vi "KeithleyInit.vi"(8 "Bottom Coil (mA)":dbl, 9 "Top Coil (mA)":dbl, 11 "KeithleyVISA In":refnum<visa-resource-name>) -> (0 "error out":errorcluster, 2 "Node Out":string, 3 "KeithleyVISA Out":refnum<visa-resource-name>)   [LabVIEW 2018]
uses:
  Channel.ctl
  Keithley 2600 Series.lvlib
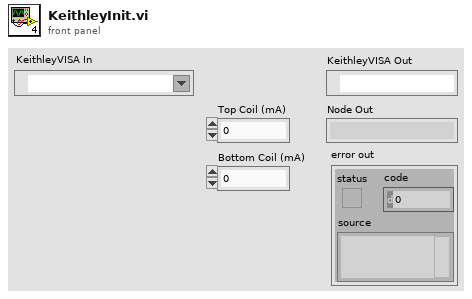
[diagram p1: front panel]
types:
  T1 = typedef "Keithley 2600 Series.lvlib/Channel.ctl" = enum32{"Channel A", "Channel B"}
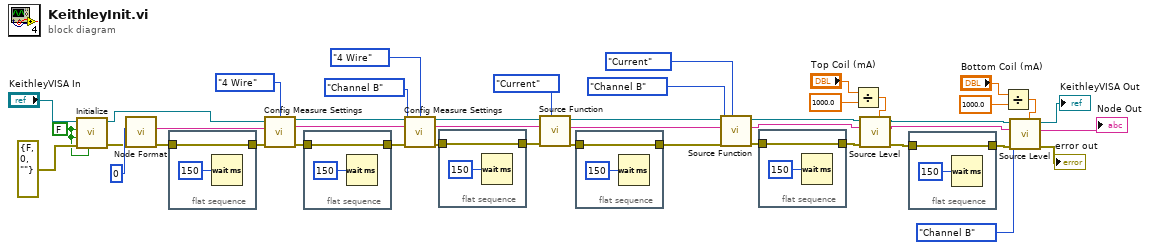
[diagram p0: block diagram]
diagram:
  w19 = FALSE ("ID Query (True)")
  n1 = call "Initialize.vi"("Reset (True)"=w19, "error in (no error)"=errorcluster {"status"=FALSE, "code"=0, "source"=""}, "Error Query (False)"=w19, "ID Query (True)"=w19, "VISA resource name"="KeithleyVISA In") -> ("error out"=w21:errorcluster, "VISA resource name out"=w22:refnum<visa-resource-name>)  [unwired: 5 in]
  n2 = call "Node Format.vi"("error in"=w21, "Node (0-64)"=i8 0) -> ("error out"=w31:errorcluster, "Formatted Node"=w36:string)  [unwired: 8 in]
  n3 = flat-sequence {
    tunnel: w31 -> [w46]
    tunnel: [w46] -> w30
    frame #0 {
      n4 = Wait (ms)(milliseconds to wait=u32 150) -> ()  [unwired: 1 out]
    }
  }
  n5 = call "Config Measure Settings.vi"("VISA resource name"=w22, "Sense (2 Wire)"=enum32{"2 Wire", "4 Wire", "Calibration"}."4 Wire", "Node In"=w36, "error in"=w30) -> ("VISA resource name out"=w43:refnum<visa-resource-name>, "Node Out"=w35:string, "error out"=w29:errorcluster)  [unwired: 8 in, 1 out]
  n6 = flat-sequence {
    tunnel: w29 -> [w48]
    tunnel: [w48] -> w28
    frame #0 {
      n7 = Wait (ms)(milliseconds to wait=u32 150) -> ()  [unwired: 1 out]
    }
  }
  n8 = call "Config Measure Settings.vi"("VISA resource name"=w43, "Sense (2 Wire)"=enum32{"2 Wire", "4 Wire", "Calibration"}."4 Wire", "Node In"=w35, "Channel (Channel A)"=Channel."Channel B", "error in"=w28) -> ("VISA resource name out"=w42:refnum<visa-resource-name>, "Node Out"=w34:string, "error out"=w27:errorcluster)  [unwired: 7 in, 1 out]
  n9 = flat-sequence {
    tunnel: w27 -> [w50]
    tunnel: [w50] -> w26
    frame #0 {
      n10 = Wait (ms)(milliseconds to wait=u32 150) -> ()  [unwired: 1 out]
    }
  }
  n11 = call "Source Function.vi"("Function (Current)"=enum32{"Current", "Voltage"}."Current", "error in (no error)"=w26, "Node In"=w34, "VISA resource name"=w42) -> ("error out"=w25:errorcluster, "Node Out"=w33:string, "VISA resource name out"=w41:refnum<visa-resource-name>)  [unwired: 4 in, 1 out]
  n12 = flat-sequence {
    tunnel: w25 -> [w52]
    tunnel: [w52] -> w24
    frame #0 {
      n13 = Wait (ms)(milliseconds to wait=u32 150) -> ()  [unwired: 1 out]
    }
  }
  n14 = call "Source Function.vi"("Function (Current)"=enum32{"Current", "Voltage"}."Current", "error in (no error)"=w24, "Channel (Channel A)"=Channel."Channel B", "Node In"=w33, "VISA resource name"=w41) -> ("error out"=w18:errorcluster, "Node Out"=w15:string, "VISA resource name out"=w16:refnum<visa-resource-name>)  [unwired: 3 in, 1 out]
  n15 = flat-sequence {
    tunnel: w18 -> [w54]
    tunnel: [w54] -> w17
    frame #0 {
      n16 = Wait (ms)(milliseconds to wait=u32 150) -> ()  [unwired: 1 out]
    }
  }
  n17 = Divide(x="Top Coil (mA)", y=1000.0) -> (x/y=w12:dbl)
  n18 = call "Source Level.vi"("Level (0.000)"=w12, "error in (no error)"=w17, "Node In"=w15, "VISA resource name"=w16) -> ("error out"=w7:errorcluster, "Node Out"=w5:string, "VISA resource name out"=w6:refnum<visa-resource-name>)  [unwired: 4 in, 1 out]
  n19 = flat-sequence {
    tunnel: w7 -> [w56]
    tunnel: [w56] -> w11
    frame #0 {
      n20 = Wait (ms)(milliseconds to wait=u32 150) -> ()  [unwired: 1 out]
    }
  }
  n21 = Divide(x="Bottom Coil (mA)", y=1000.0) -> (x/y=w8:dbl)
  n22 = call "Source Level.vi"("Level (0.000)"=w8, "error in (no error)"=w11, "Channel (Channel A)"=Channel."Channel B", "Node In"=w5, "VISA resource name"=w6) -> ("error out"=→"error out":errorcluster, "Node Out"=→"Node Out":string, "VISA resource name out"=→"KeithleyVISA Out":refnum<visa-resource-name>)  [unwired: 3 in, 1 out]
